vi "Do.vi"(8 "error in (no error)":errorcluster, 10 "Actor in":refnum<class "Actor.lvclass">, 11 "DeInit Done Msg":refnum<class "DeInit Done Msg.lvclass">) -> (0 "error out":errorcluster, 2 "Actor out":refnum<class "Actor.lvclass">)   [LabVIEW 2023, in "InitDeInit.lvlib" / "DeInit Done Msg.lvclass"]
doc: "This VI delivers the message to the actor by calling the appropriate method(s) on the actor."
uses:
  DeInit Done Msg.lvclass
  89ad2160-1e8c-49df-ae49-c8cdb6330e83.vi
  InitDeinitComm/InitDeinitComm.lvclass
  <vilib>/ActorFramework/Actor/Actor.lvclass
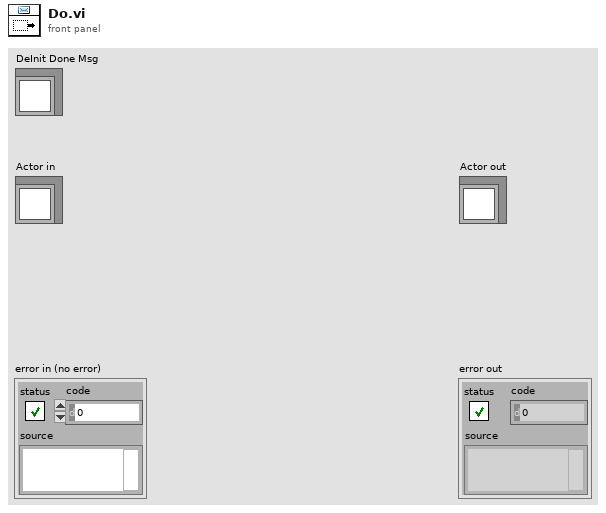
[diagram p1: front panel]
types:
  T1 = typedef "typedefs.lvlib/InstrumentData.ctl" = cluster{"Instr Error":errorcluster, "Address":cluster{"address type":enum16{"VISA", "Index"}, "Address":string, "instrument type":T2}, "CurrentState":cluster{"Initialized":bool, "Connected":bool, "Running":bool, "Error":bool}}
  T2 = typedef "typedefs.lvlib/instrumentType.ctl" = enum16{"Spectrometer", "Camera", "Stepper", "Piezo"}
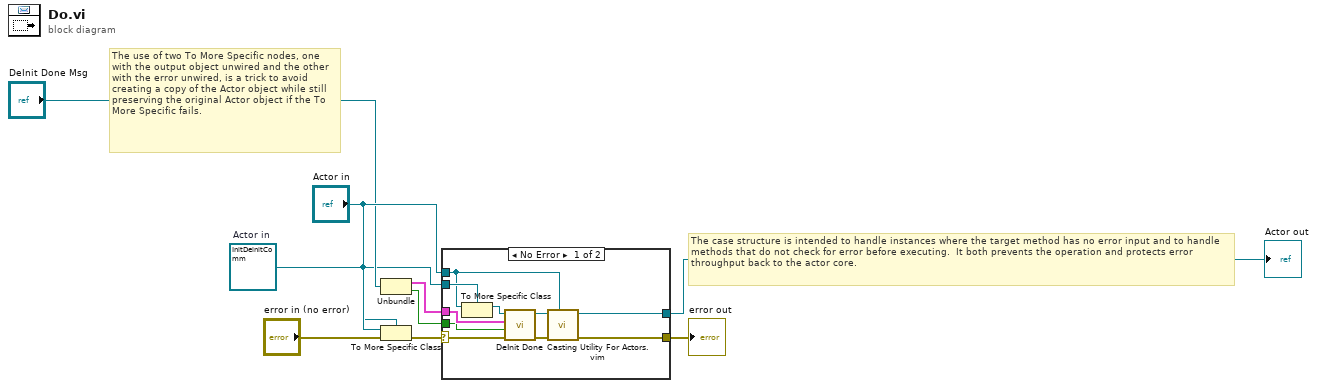
[diagram p0: block diagram]
diagram:
  w4 = refnum<class "InitDeinitComm.lvclass"> refnum  # Actor in
  # "The use of two To More Specific nodes, one with the output object unwired and the other with the error unwired, is a trick to avoid creating a copy of the Actor object while still preserving the original Actor object if the To More Specific fails."
  # "The case structure is intended to handle instances where the target method has no error input and to handle methods that do not check for error before executing.  It both prevents the operation and protects error throughput back to the actor core."
  n1 = Unbundle("DeInit Done Msg") -> (w2:T1, w1:bool)
  n2 = To More Specific Class(target class=w4, reference="Actor in", error in="error in (no error)") -> (error out=w3:errorcluster)  [unwired: 1 out]
  n3 = case shown="No Error" w3 {
    selector: w3 -> [w19 w21]
    tunnel: [w13 w21] -> w9
    tunnel: [w14 w20] -> w8
    tunnel: "Actor in" -> [w16 w20]
    tunnel: w4 -> [w17 _]
    tunnel: w2 -> [w11 _]
    tunnel: w1 -> [w10 _]
    frame No Error {
      n4 = To More Specific Class(target class=w17, reference=w16) -> (specific class reference=w18:refnum<class "InitDeinitComm.lvclass">)  [unwired: 1 in, 1 out]
      n5 = call-dynamic "DeInit Done.vi"("error in (no error)"=w19, "Initialized"=w10, "InstrumentData"=w11, "InitDeinitComm.lvclass"=w18) -> ("error out"=w12:errorcluster, "InitDeinitComm.lvclass"=w15:refnum<class "InitDeinitComm.lvclass">)  [unwired: 6 in]
      n6 = call "Casting Utility For Actors.vim"("type"=w16, "error in (no error)"=w12, "Actor in"=w15) -> ("error out"=w13:errorcluster, "Actor out"=w14:refnum<class "Actor.lvclass">)  [unwired: 7 in]
    }
    frame Error {
      # "If type check fails, pass the original object out again."
    }
  }
  "error out" <- w9
  "Actor out" <- w8
